vi "MDF4 Create File.vi"(7 "Error In":errorcluster, 9 "History":T1={"History"="my History", "ID"="LabVIEW Logger", "Vendor"="National Instruments", "Version"="1.0"}, 10 "MDF4 File Path":path) -> (0 "Error Out":errorcluster, 3 "MDF4 File Reference out":i64)   [LabVIEW 2019, in "MD4Logger Engine.lvlib"]
uses:
  MD4Logger Engine.lvlib
  <vilib>/Utility/error.llb/Error Cluster From Error Code.vi
  <vilib>/ErrorRing/Error Ring.xnode
  <vilib>/NI VeriStand/Custom Device Tools/Custom Device Utility Library/Custom Device Utility Library.lvlib
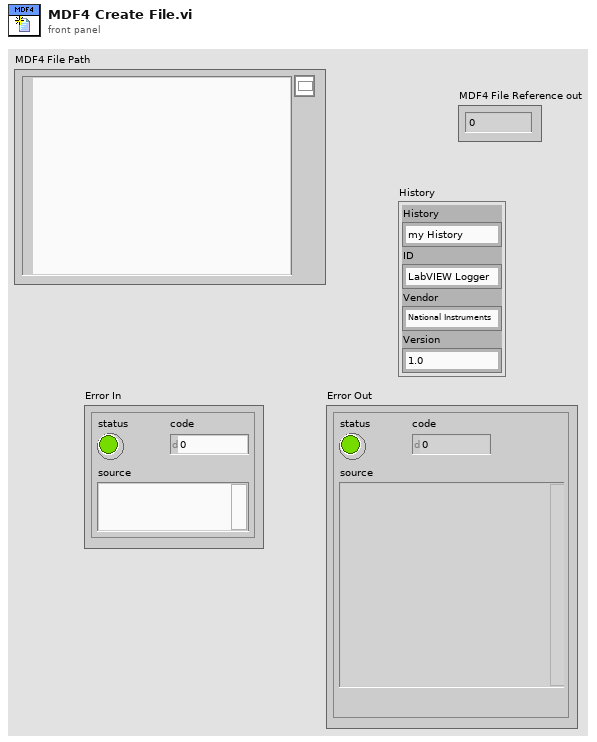
[diagram p1: front panel]
types:
  T1 = cluster{"History":string, "ID":string, "Vendor":string, "Version":string}
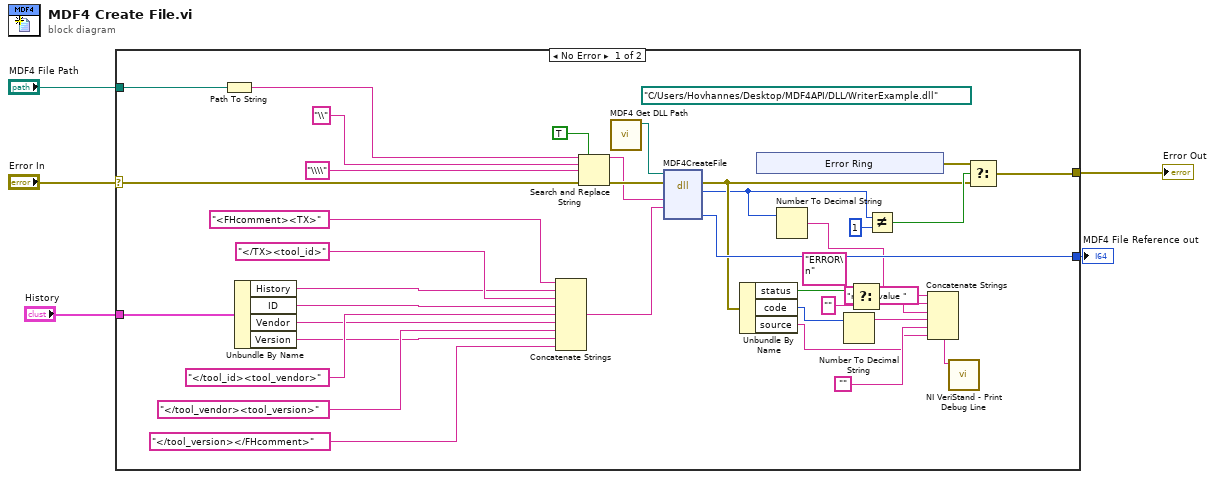
[diagram p0: block diagram]
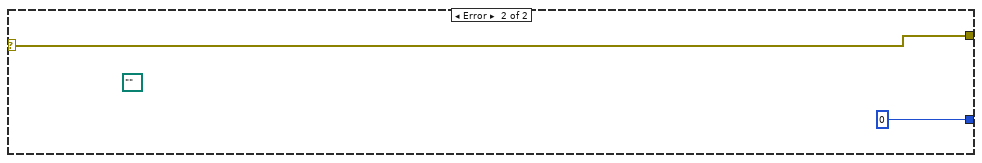
[diagram p2: hidden frame]
diagram:
  n1 = case shown="No Error" "Error In" {
    selector: "Error In" -> [w24 w50]
    tunnel: [w30 w50] -> w4
    tunnel: "MDF4 File Path" -> [w43 _]
    tunnel: [w42 i64 0 ("pFileWriter")] -> w2
    tunnel: "History" -> [w35 _]
    frame No Error {
      (unwired) path "C:/Users/Hovhannes/Desktop/MDF4API/DLL/WriterExample.dll" ("path in")
      n2 = Path To String(path=w43) -> (string=w27:string)
      n3 = Unbundle By Name(w35) -> ("History"=w34:string, "ID"=w33:string, "Vendor"=w32:string, "Version"=w31:string)
      n4 = Concatenate Strings("<FHcomment><TX>", w34, "</TX><tool_id>", w33, "</tool_id><tool_vendor>", w32, "</tool_vendor><tool_version>", w31, "</tool_version></FHcomment>") -> (w38:string)
      n5 = Search and Replace String(replace all?=TRUE ("replace all? (F)"), input string=w27, search string="\\", replace string="\\\\", error in=w24) -> (result string=w22:string, error out=w23:errorcluster)  [unwired: 3 in, 2 out]
      n6 = call "MDF4 Get DLL Path.vi"() -> ("DLL Path Out"=w6:path)  [unwired: 10 in, 1 out]
      n7 = dll-call lib="C:/Users/Hovhannes/Desktop/MDF4API/DLL/WriterExample.dll" fn="MDF4CreateFile"(path in=w6, error in=w23, "path"=w22, "file_history"=w38) -> (error out=w19:errorcluster, "return type"=w10:i32, "m4"=w42:i64)  [unwired: 4 in, 1 out]
      n8 = Unbundle By Name(w19) -> ("status"=w18:bool, "code"=w15:i32, "source"=w12:string)
      n9 = xnode "Error Ring"() -> ("error out"=w29:errorcluster)
      n10 = Number To Decimal String(number=w10) -> (decimal integer string=w9:string)  [unwired: 1 in]
      n11 = Number To Decimal String(number=w15) -> (decimal integer string=w14:string)  [unwired: 1 in]
      n12 = Select(t="ERROR\n", s=w18, f="") -> (s? t:f=w16:string)
      n13 = Not Equal?(x=w10, y=1) -> (x != y?=w21:bool)
      n14 = Concatenate Strings("return value " ("string"), w9, w16, w14, "", w12) -> (w7:string)
      n15 = call <vilib>:"NI VeriStand - Print Debug Line.vi"("Message"=w7) -> ()  [unwired: 10 in, 1 out]
      n16 = Select(t=w29, s=w21, f=w19) -> (s? t:f=w30:errorcluster)
    }
    frame Error {
      (unwired) path "" ("path out")
    }
  }
  "MDF4 File Reference out" <- w2
  "Error Out" <- w4
